vi "MotorControl FPGA.vi"() -> ()   [LabVIEW 2013]
uses:
  <vilib>/eio/EIONode/EIONode.xnode
  <vilib>/rvi/eio/common/nirviEmuTemplateMethod_errors.vi
panel:
  in  "Knob":i16(knob) scale=0.0..100.0
  in  "Boolean":bool
  in  "Cluster":cluster{"Pulse Period (Ticks)":i16}
  in  "Enable":bool
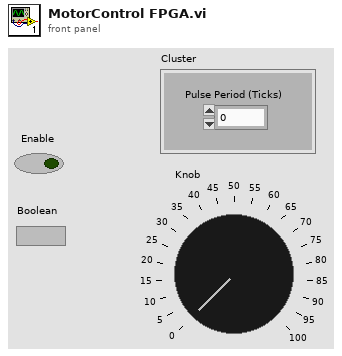
[diagram p1: front panel]
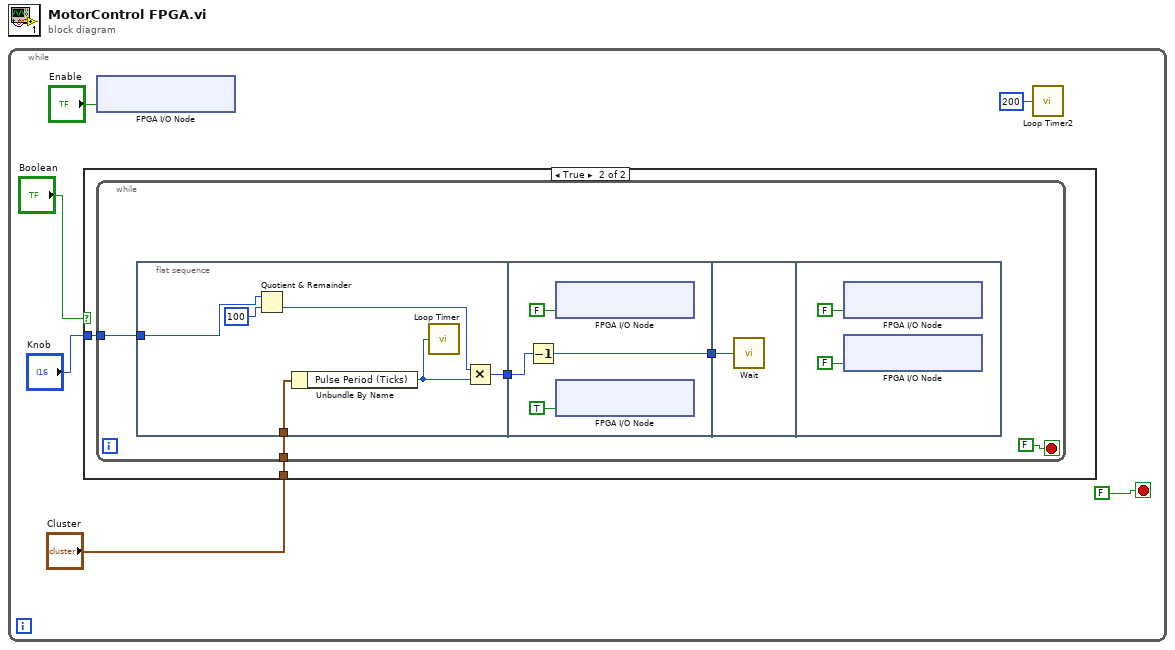
[diagram p0: block diagram]
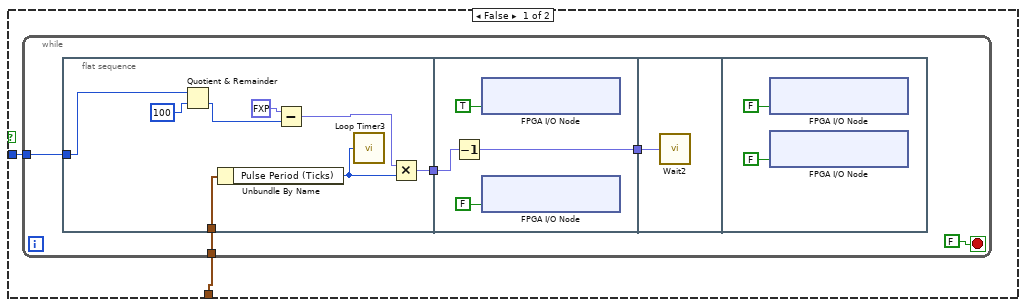
[diagram p2: hidden frame]
diagram:
  n1 = while {
    stop <- FALSE stop-if-true
    n2 = case shown="True" "Boolean" {
      tunnel: "Knob" -> [w7 w30]
      tunnel: "Cluster" -> [w8 w29]
      frame False {
        n3 = while {
          tunnel: w8 -> [w10]
          tunnel: w7 -> [w9]
          stop <- FALSE stop-if-true
          n4 = flat-sequence {
            tunnel: [w21] -> w11
            tunnel: w10 -> [w15]
            tunnel: w9 -> [w14]
            tunnel: [w24] -> w13
            tunnel: w11 -> [w22]
            tunnel: w13 -> [w26]
            frame #0 {
              n5 = Quotient & Remainder(x=w14, y=i16 100) -> (floor(x/y)=w17:i16)  [unwired: 1 out]
              n6 = Unbundle By Name(w15) -> ("Pulse Period (Ticks)"=w19:i16)
              n7 = Subtract(x=fxp<+,1,1> 1.0, y=w17) -> (x-y=w16:fxp<+/-,17,17>)
              n8 = call "Loop Timer3"("Count(Ticks)"=w19) -> ()  [unwired: 1 out]
              n9 = Multiply(x=w16, y=w19) -> (x*y=w21:fxp<+/-,32,32>)
            }
            frame #1 {
              n10 = Decrement(x=w22) -> (x-1=w24:fxp<+/-,32,32>)
              n11 = xnode "FPGA I/O Node"("ConnectorC/DIO7"=TRUE) -> ()  [unwired: 1 in, 1 out]
              n12 = xnode "FPGA I/O Node"("ConnectorC/DIO3"=FALSE ("ConnectorC/DIO7")) -> ()  [unwired: 1 in, 1 out]
            }
            frame #2 {
              n13 = call "Wait2"("Count(Ticks)"=w26) -> ()  [unwired: 1 out]
            }
            frame #3 {
              n14 = xnode "FPGA I/O Node"("ConnectorC/DIO7"=FALSE) -> ()  [unwired: 1 in, 1 out]
              n15 = xnode "FPGA I/O Node"("ConnectorC/DIO3"=FALSE ("ConnectorC/DIO7")) -> ()  [unwired: 1 in, 1 out]
            }
          }
        }
      }
      frame True {
        n16 = while {
          tunnel: w30 -> [w32]
          tunnel: w29 -> [w31]
          stop <- FALSE stop-if-true
          n17 = flat-sequence {
            tunnel: [w41] -> w33
            tunnel: w32 -> [w37]
            tunnel: w31 -> [w36]
            tunnel: [w44] -> w35
            tunnel: w33 -> [w42]
            tunnel: w35 -> [w46]
            frame #0 {
              n18 = Quotient & Remainder(x=w37, y=i16 100) -> (floor(x/y)=w38:i16)  [unwired: 1 out]
              n19 = Unbundle By Name(w36) -> ("Pulse Period (Ticks)"=w40:i16)
              n20 = call "Loop Timer"("Count(Ticks)"=w40) -> ()  [unwired: 1 out]
              n21 = Multiply(x=w38, y=w40) -> (x*y=w41:i16)
            }
            frame #1 {
              n22 = Decrement(x=w42) -> (x-1=w44:i16)
              n23 = xnode "FPGA I/O Node"("ConnectorC/DIO7"=FALSE) -> ()  [unwired: 1 in, 1 out]
              n24 = xnode "FPGA I/O Node"("ConnectorC/DIO3"=TRUE ("ConnectorC/DIO7")) -> ()  [unwired: 1 in, 1 out]
            }
            frame #2 {
              n25 = call "Wait"("Count(Ticks)"=w46) -> ()  [unwired: 1 out]
            }
            frame #3 {
              n26 = xnode "FPGA I/O Node"("ConnectorC/DIO7"=FALSE) -> ()  [unwired: 1 in, 1 out]
              n27 = xnode "FPGA I/O Node"("ConnectorC/DIO3"=FALSE ("ConnectorC/DIO7")) -> ()  [unwired: 1 in, 1 out]
            }
          }
        }
      }
    }
    n28 = xnode "FPGA I/O Node"("ConnectorA/DIO0"="Enable") -> ()  [unwired: 1 in, 1 out]
    n29 = call "Loop Timer2"("Count(mSec)"=u32 200) -> ()  [unwired: 1 out]
  }
